vi "写配置参数.vi"(8 "error in (no error)":errorcluster caption="错误输入（无错误）", 10 "values":u16[](array[numeric]), 11 "参数":enum16{"氨氮", "总磷", "总氮", "CODMn", "CODcr"}(ring)) -> (0 "error out":errorcluster caption="错误输出")   [LabVIEW 2016]
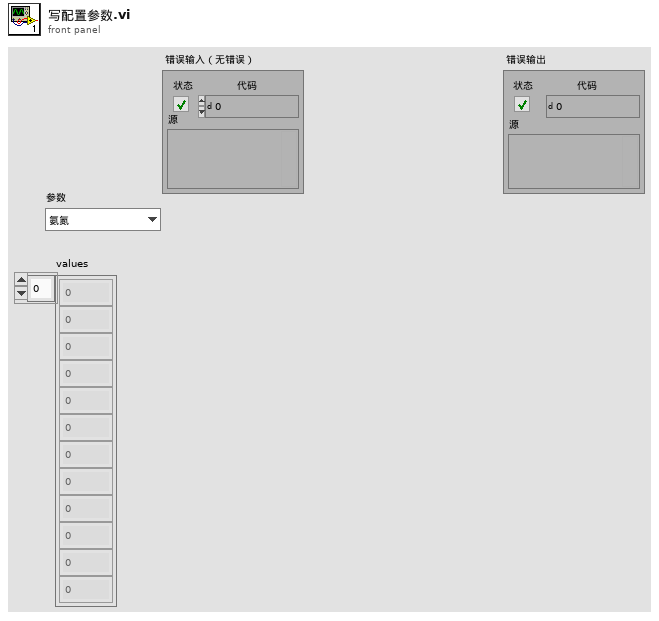
[diagram p1: front panel]
types:
  T1 = cluster{"氨氮":u8, "总磷":u8, "总氮":u8, "CODMn":u8, "CODCr":u8}
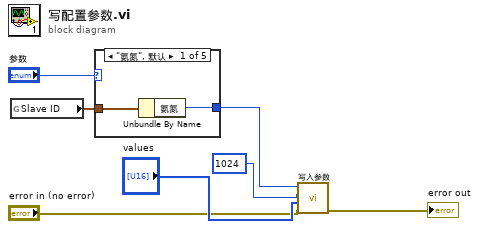
[diagram p0: block diagram]
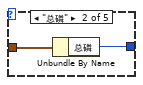
[diagram p2: hidden frame]
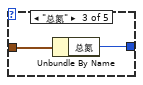
[diagram p3: hidden frame]
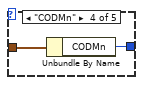
[diagram p4: hidden frame]
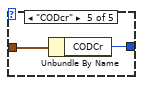
[diagram p5: hidden frame]
diagram:
  n1 = global read "断电保存全局.vi" "Slave ID"() -> (w7:T1)
  n2 = case shown="\"氨氮\", 默认" "参数" {
    tunnel: w7 -> [w9 w11 w13 w15 w17]
    tunnel: [w8 w10 w12 w14 w16] -> w5
    frame "氨氮", Default {
      n3 = Unbundle By Name(w9) -> ("氨氮"=w8:u8)
    }
    frame "总磷" {
      n4 = Unbundle By Name(w11) -> ("总磷"=w10:u8)
    }
    frame "总氮" {
      n5 = Unbundle By Name(w13) -> ("总氮"=w12:u8)
    }
    frame "CODMn" {
      n6 = Unbundle By Name(w15) -> ("CODMn"=w14:u8)
    }
    frame "CODcr" {
      n7 = Unbundle By Name(w17) -> ("CODCr"=w16:u8)
    }
  }
  n8 = call "写入参数.vi"("Error in"="error in (no error)", "values"="values", "starting address"=u16 1024, "Slave ID"=w5) -> ("error out"=→"error out":errorcluster)  [unwired: 7 in]
